vi "CB Serial Test.vi"(8 "error in (no error)":errorcluster) -> (0 "error out":errorcluster, 1 "Pass/Fail":bool, 2 "VISA resource OUT":refnum<visa-resource-name>, 3 "Actual Result":string, 7 "Expected Result":string)   [LabVIEW 2022 SP3]
uses:
  <vilib>/Instr/_visa.llb/VISA Flush IO Buffer Mask.ctl
panel:
  out "output string":string
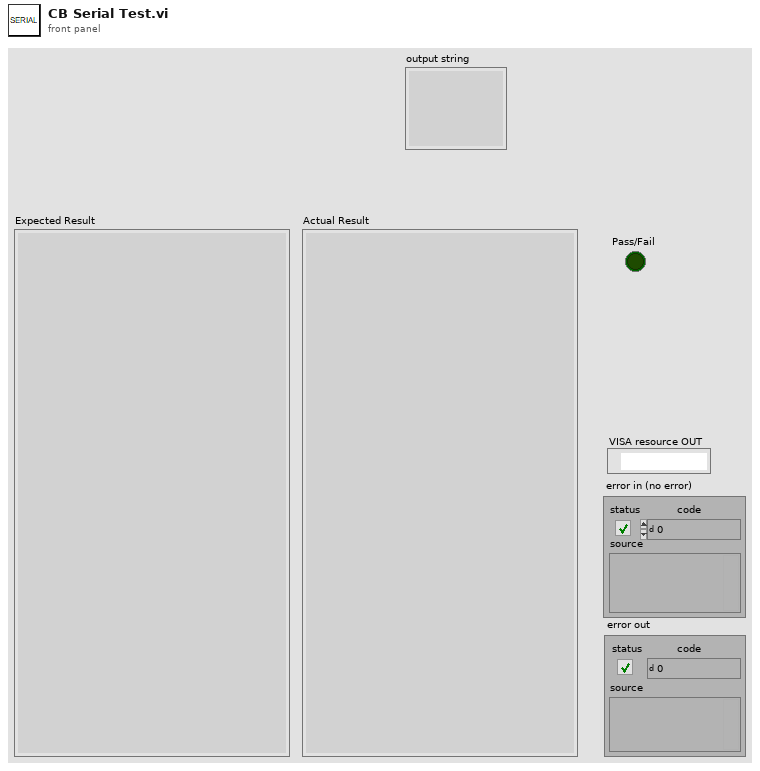
[diagram p1: front panel]
types:
  T1 = typedef "VISA Flush IO Buffer Mask.ctl" = u16
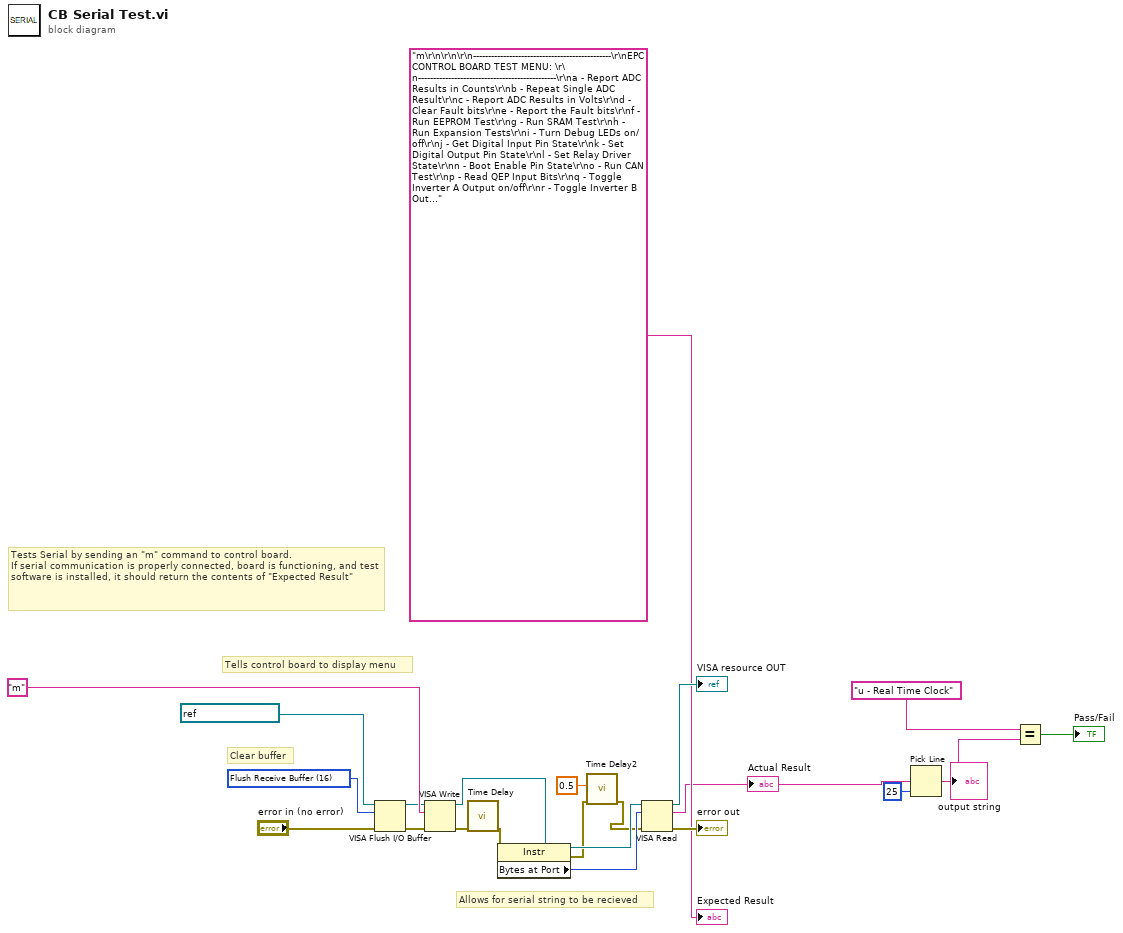
[diagram p0: block diagram]
diagram:
  w19 = T1 16 items=["Flush Receive Buffer"=16, "Write Transmit Buffer to Device"=32, "Flush Receive Buffer (No I/O)"=64, "Flush Transmit Buffer"=128] ("Mask")
  # "Tests Serial by sending an \"m\" command to control board.\nIf serial communication is properly connected, board is functioning, and test software is installed, it should return the contents of \"Expected Result\""
  # "Clear buffer"
  # "Allows for serial string to be recieved"
  # "Tells control board to display menu"
  n1 = VISA Flush I/O Buffer(VISA resource name=refnum<visa-resource-name> "ControlBoard", mask (16)=w19, error in (no error)="error in (no error)") -> (VISA resource name out=w17:refnum<visa-resource-name>, error out=w16:errorcluster)
  n2 = VISA Write(VISA resource name=w17, write buffer="m", error in (no error)=w16) -> (VISA resource name out=w14:refnum<visa-resource-name>, error out=w18:errorcluster)  [unwired: 1 out]
  n3 = call "Time Delay"("error in (no error)"=w18) -> ("error out"=w15:errorcluster)  [unwired: 10 in]
  n4 = property class="Instr"(reference=w14, error in=w15) -> (reference out=w21:refnum<visa-resource-name>, error out=w8:errorcluster, "Bytes at Port"=w20:u32)
  n5 = call "Time Delay2"("error in (no error)"=w8, "Delay Time (s)"=0.5) -> ("error out"=w7:errorcluster)  [unwired: 9 in]
  n6 = VISA Read(VISA resource name=w21, byte count=w20, error in (no error)=w7) -> (VISA resource name out=→"VISA resource OUT":refnum<visa-resource-name>, read buffer=w4:string, error out=→"error out":errorcluster)  [unwired: 1 out]
  "Actual Result" <- w4
  n7 = Pick Line(multi-line string=w4, line index=25) -> (output string=w1:string)  [unwired: 1 in]
  "output string" <- w1
  n8 = Equal?(x="u - Real Time Clock", y=w1) -> (x = y?=→"Pass/Fail":bool)
  "Expected Result" <- "m\r\n\r\n\r\n----------------------------------------------\r\nEPC CONTROL BOARD TEST MENU: \r\n----------------------------------------------\r\na - Report ADC Results in Counts\r\nb - Repeat Single ADC Result\r\nc - Report ADC Results in Volts\r\nd - Clear Fault bits\r\ne - Report the Fault bits\r\nf - Run EEPROM Test\r\ng - Run SRAM Test\r\nh - Run Expansion Tests\r\ni - Turn Debug LEDs on/off\r\nj - Get Digital Input Pin State\r\nk - Set Digital Output Pin State\r\nl - Set Relay Driver State\r\nn - Boot Enable Pin State\r\no - Run CAN Test\r\np - Read QEP Input Bits\r\nq - Toggle Inverter A Output on/off\r\nr - Toggle Inverter B Output on/off\r\ns - Toggle Half Bridge Output on/off\r\nt - Set PWM leg duty cycle\r\nu - Real Time Clock\r\nv - Watchdog Control\r\nw - Test Interrupt Lines\r\nx - Read HALLs\r\ny - Test FPGA Read/Write\r\nz - Report Software/FPGA Revs\r\nm - Display this menu\r\n0 - Report Internal RAM Zeroed\r\n1 - Report SRAM Zeroed\r\n2 - Report SRAM Initialized\r\n3 - Run Quick EEPROM Test\r\n4 - Report Temperature and Humidity\r\n> "
